vi "niDTS WLAN Tx Test UTIL Parameters to DUT Parameters.vi"(7 "Parameters":T1={"Standard"=enum."802.11 n HT", "DSSS Data Rate (Mbps)"=enum."1", "OFDM Data Rate (Mbps)"=enum."54", "MCS Index"=7, "N spatial streams"=1, "Chains"=[TRUE, FALSE, FALSE, FALSE], "BandWidth (Hz)"=enum."20 MHz", "Channel"=0, "Gard Interval"=enum."SHORT", "FEC Coding"=enum."LDPC", "Dut Tx Power"=1.0, "16 symbols"=TRUE, "payload length bytes"=1500, "idle interval"=0.0001, "External Attenuation"=[0.0, 0.0, 0.0, 0.0], "Acquisition Parameters "={"Acquisition Length Mode"=enum."AUTO", "Acquisition Length (s)"=0.00015, "Auto Level"=FALSE}, "TXP Measurement Parameters"={"TXP Power Enable"=TRUE, "TXP Averages"=3}, "ModAcc Measurement Paramaters"={"ModAcc Enable"=FALSE, "Header Detection"=enum."MANUAL", "Averages"=3, "Amplitude Tracking"=FALSE, "Channel Tracking"=FALSE, "Time Tracking"=TRUE, "Phase Tracking"=enum."NONE", "Clock Offset Est"=FALSE, "Impairments Est"=FALSE, "CFO Estimation"=enum."PAMBLE"}, "ModAcc DSSS Paramaters"={"DC Offset Compensation"=TRUE, "Equalization"=TRUE, "Phase Tracking"=TRUE, "Chip Start Location"=0, "Max Chips Used"=16, "Pulse Shaping FilterType"=enum."GAUSSIAN", "Pulse Shaping Filter Coefficient"=0.35}, "SEM Measurement Parameters"={"SEM Enable"=TRUE, "SEM Averages"=3, "Auto Span Enable"=TRUE, "Frequency Span (Hz)"=66000000.0, "Measurement Type"=enum."Standard", "Mask Frequencies (Hz)"=[], "Mask Power Offsets (dB)"=[]}, "OBW Measurement Parameters"={"OBW Enable"=FALSE, "OBW Averages"=3}, "DSSS Power Ramp"={"Power Ramp Enable"=FALSE, "Averages"=3, "Thresholds"={"Up Low (%)"=10.0, "Down Low (%)"=10.0, "Up High (%)"=90.0, "Down High (%)"=90.0}}, "Enable Traces"=FALSE} {"DSSS Power Ramp"."Thresholds"."Down High (%)" min=0.0 max=100.0 step=1.0; "DSSS Power Ramp"."Thresholds"."Up High (%)" min=0.0 max=100.0 step=1.0; "DSSS Power Ramp"."Thresholds"."Down Low (%)" min=0.0 max=100.0 step=1.0; "DSSS Power Ramp"."Thresholds"."Up Low (%)" min=0.0 max=100.0 step=1.0; "Acquisition Parameters"."Acquisition Length (s)" format="%#_6p"; "SEM Measurement Parameters"."Frequency Span (Hz)" format="%#_6p"; "idle interval" format="%_3p"}) -> (8 "TV Parameters(DataType)":T16={"WLAN Type"=enum."b - 1 Mbps", "Bandwidth (Hz)"=enum."20 MHz", "Channel"=0, "Guard Interval"=enum."LONG", "FEC Coding"=enum."LDPC", "Power (dBm)"=0.0, "Payload Length (bytes)"=1500, "16 Symbols"=TRUE, "Chains"=[TRUE, FALSE, FALSE, FALSE]})   [LabVIEW 2015, in "niDTS WLAN.lvlib"]
uses:
  niDTS WLAN.lvlib
  Includes/niDTS WLAN DUT INC Parameters.ctl
  Includes/niDTS WLAN INC Type.ctl
  Includes/niDTS WLAN INC CH BW.ctl
  Includes/niDTS WLAN INC GI.ctl
  Includes/niDTS WLAN INC FEC Coding.ctl
  Includes/niDTS WLAN Tx Test INC Parameters.ctl
  Includes/niDTS WLAN INC Standard.ctl
  Includes/niDTS WLAN INC DSSS Data Rate.ctl
  Includes/niDTS WLAN INC OFDM Data Rate.ctl
  Includes/niDTS WLAN DUT INC Acquisition Parameters.ctl
  Includes/niDTS WLAN INC TXP Measurement Parameters.ctl
  Includes/niDTS WLAN INC ModAcc Measurement Parameters.ctl
  Includes/niDTS WLAN INC DSSS ModAcc Measurement Parameters.ctl
  Includes/niDTS WLAN INC Pulse Shaping Filter Type.ctl
  Includes/niDTS WLAN INC SEM Measurement Parameters.ctl
  Includes/niDTS WLAN INC OBW Measurement Parameters.ctl
  Includes/niDTS WLAN INC DSSS Power Ramp Parameters.ctl
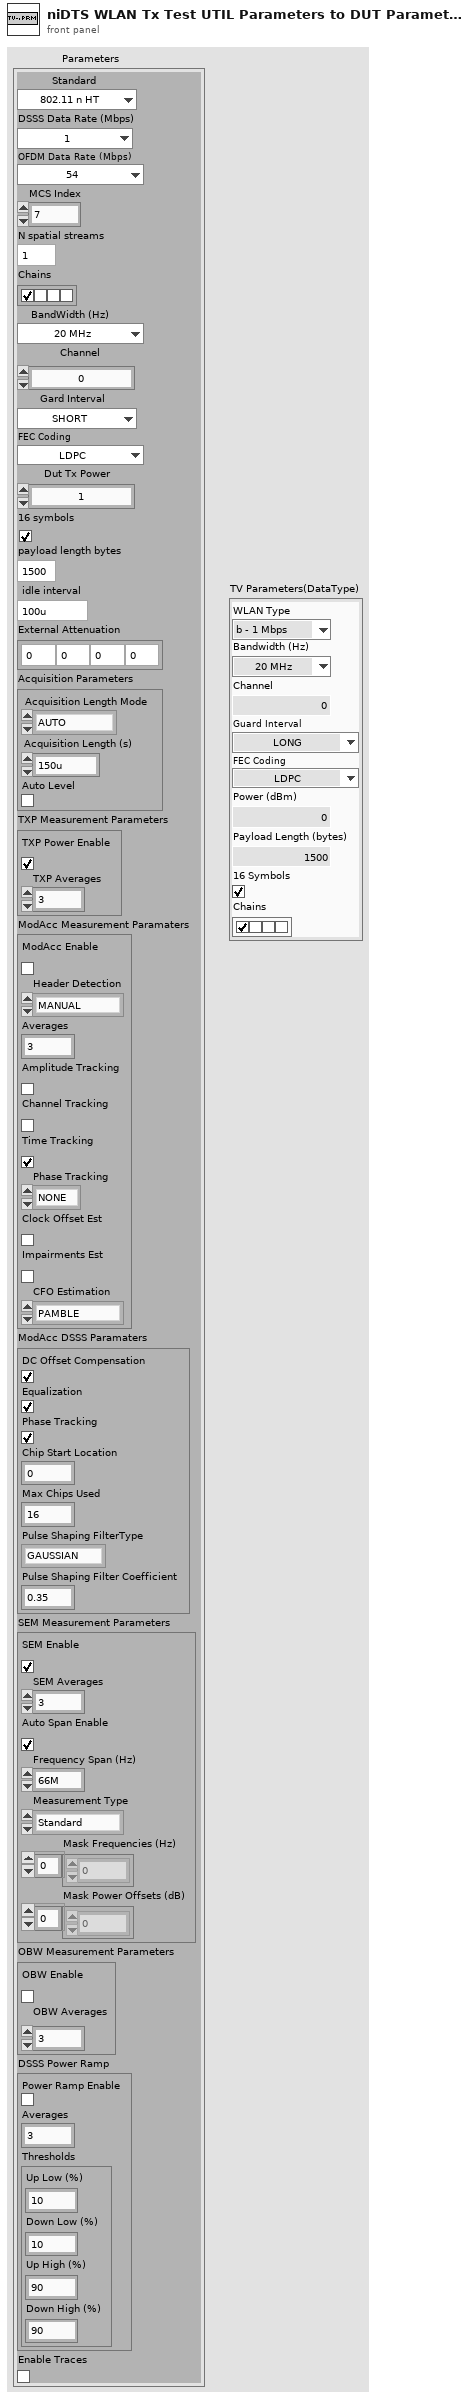
[diagram p1: front panel]
types:
  T1 = typedef "niDTS WLAN.lvlib/niDTS WLAN Tx Test INC Parameters.ctl" = cluster{"Standard":T2, "DSSS Data Rate (Mbps)":T3, "OFDM Data Rate (Mbps)":T4, "MCS Index":i32, "N spatial streams":i32, "Chains":bool[], "BandWidth (Hz)":T5, "Channel":i32, "Gard Interval":T6, "FEC Coding":T7, "Dut Tx Power":dbl, "16 symbols":bool, "payload length bytes":i32, "idle interval":dbl, "External Attenuation":dbl[], "Acquisition Parameters ":T8, "TXP Measurement Parameters":T9, "ModAcc Measurement Paramaters":T10, "ModAcc DSSS Paramaters":T11, "SEM Measurement Parameters":T13, "OBW Measurement Parameters":T14, "DSSS Power Ramp":T15, "Enable Traces":bool}
  T2 = typedef "niDTS WLAN.lvlib/niDTS WLAN INC Standard.ctl" = enum16{"802.11 b DSSS", "802.11 a/g OFDM", "802.11 n HT", "802.11 ac VHT"}
  T3 = typedef "niDTS WLAN.lvlib/niDTS WLAN INC DSSS Data Rate.ctl" = enum16{"1", "2", "5.5", "11"}
  T4 = typedef "niDTS WLAN.lvlib/niDTS WLAN INC OFDM Data Rate.ctl" = enum16{"6", "9", "12", "18", "24", "36", "48", "54"}
  T5 = typedef "niDTS WLAN.lvlib/niDTS WLAN INC CH BW.ctl" = enum16{"20 MHz", "40 MHz", "80 MHz", "160 MHz"}
  T6 = typedef "niDTS WLAN.lvlib/niDTS WLAN INC GI.ctl" = enum16{"LONG", "SHORT"}
  T7 = typedef "niDTS WLAN.lvlib/niDTS WLAN INC FEC Coding.ctl" = enum16{"BCC", "LDPC"}
  T8 = typedef "niDTS WLAN.lvlib/niDTS WLAN DUT INC Acquisition Parameters.ctl" = cluster{"Acquisition Length Mode":enum16{"AUTO", "MANUAL"}, "Acquisition Length (s)":dbl, "Auto Level":bool}
  T9 = typedef "niDTS WLAN.lvlib/niDTS WLAN INC TXP Measurement Parameters.ctl" = cluster{"TXP Power Enable":bool, "TXP Averages":i32}
  T10 = typedef "niDTS WLAN.lvlib/niDTS WLAN INC ModAcc Measurement Parameters.ctl" = cluster{"ModAcc Enable":bool, "Header Detection":enum16{"MANUAL", "FIRST", "ALL"}, "Averages":i32, "Amplitude Tracking":bool, "Channel Tracking":bool, "Time Tracking":bool, "Phase Tracking":enum16{"NONE", "STANDARD", "CSF", "INSTANT"}, "Clock Offset Est":bool, "Impairments Est":bool, "CFO Estimation":enum16{"PAMBLE", "PDATA"}}
  T11 = typedef "niDTS WLAN.lvlib/niDTS WLAN INC DSSS ModAcc Measurement Parameters.ctl" = cluster{"DC Offset Compensation":bool, "Equalization":bool, "Phase Tracking":bool, "Chip Start Location":i16, "Max Chips Used":i16, "Pulse Shaping FilterType":T12, "Pulse Shaping Filter Coefficient":dbl}
  T12 = typedef "niDTS WLAN.lvlib/niDTS WLAN INC Pulse Shaping Filter Type.ctl" = enum16{"NONE", "RCOSINE", "RRCOSINE", "GAUSSIAN"}
  T13 = typedef "niDTS WLAN.lvlib/niDTS WLAN INC SEM Measurement Parameters.ctl" = cluster{"SEM Enable":bool, "SEM Averages":i32, "Auto Span Enable":bool, "Frequency Span (Hz)":dbl, "Measurement Type":enum16{"Standard", "Legacy", "Custom"}, "Mask Frequencies (Hz)":dbl[], "Mask Power Offsets (dB)":dbl[]}
  T14 = typedef "niDTS WLAN.lvlib/niDTS WLAN INC OBW Measurement Parameters.ctl" = cluster{"OBW Enable":bool, "OBW Averages":i32}
  T15 = typedef "niDTS WLAN.lvlib/niDTS WLAN INC DSSS Power Ramp Parameters.ctl" = cluster{"Power Ramp Enable":bool, "Averages":i32, "Thresholds":cluster{"Up Low (%)":dbl, "Down Low (%)":dbl, "Up High (%)":dbl, "Down High (%)":dbl}}
  T16 = typedef "niDTS WLAN.lvlib/niDTS WLAN DUT INC Parameters.ctl" = cluster{"WLAN Type":T17, "Bandwidth (Hz)":T5, "Channel":i32, "Guard Interval":T6, "FEC Coding":T7, "Power (dBm)":dbl, "Payload Length (bytes)":i32, "16 Symbols":bool, "Chains":bool[]}
  T17 = typedef "niDTS WLAN.lvlib/niDTS WLAN INC Type.ctl" = enum16{"b - 1 Mbps", "b - 2 Mbps", "b - 5.5 Mbps", "b - 11 Mbps", "ag - 6 Mbps", "ag - 9 Mbps", "ag - 12 Mbps", "ag - 18 Mbps", "ag - 24 Mbps", "ag - 36 Mbps", "ag - 48 Mbps", "ag - 54 Mbps", "n - MCS0", "n - MCS1", "n - MCS2", "n - MCS3", "n - MCS4", "n - MCS5", "n - MCS6", "n - MCS7", "n - MCS8", "n - MCS9", "n - MCS10", "n - MCS11", "n - MCS12", "n - MCS13", "n - MCS14", "n - MCS15", "n - MCS16", "n - MCS17", "n - MCS18", "n - MCS19", "n - MCS20", "n - MCS21", "n - MCS22", "n - MCS23", "n - MCS24", "n - MCS25", "n - MCS26", "n - MCS27", "n - MCS28", "n - MCS29", "n - MCS30", "n - MCS31", "ac - MCS0 -1", "ac - MCS1 -1", "ac - MCS2 -1", "ac - MCS3 -1", "ac - MCS4 -1", "ac - MCS5 -1", "ac - MCS6 -1", "ac - MCS7 -1", "ac - MCS8 -1", "ac - MCS9 -1", "ac - MCS0 -2", "ac - MCS1 -2", "ac - MCS2 -2", "ac - MCS3 -2", "ac - MCS4 -2", "ac - MCS5 -2", "ac - MCS6 -2", "ac - MCS7 -2", "ac - MCS8 -2", "ac - MCS9 -2", "ac - MCS0 -3", "ac - MCS1 -3", "ac - MCS2 -3", "ac - MCS3 -3", "ac - MCS4 -3", "ac - MCS5 -3", "ac - MCS6 -3", "ac - MCS7 -3", "ac - MCS8 -3", "ac - MCS9 -3", "ac - MCS0 -4", "ac - MCS1 -4", "ac - MCS2 -4", "ac - MCS3 -4", "ac - MCS4 -4", "ac - MCS5 -4", "ac - MCS6 -4", "ac - MCS7 -4", "ac - MCS8 -4", "ac - MCS9 -4"}
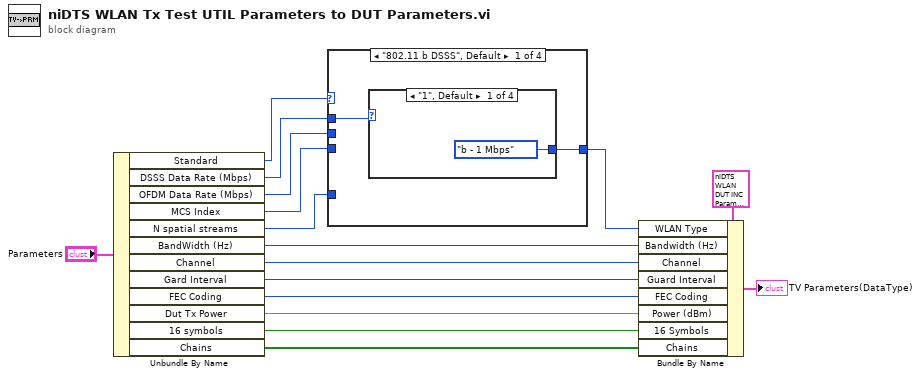
[diagram p0: block diagram]
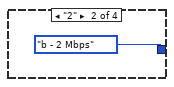
[diagram p2: hidden frame]
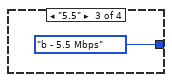
[diagram p3: hidden frame]
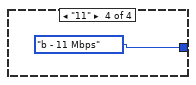
[diagram p4: hidden frame]
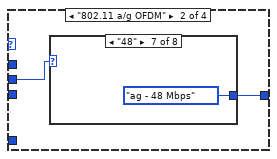
[diagram p5: hidden frame]
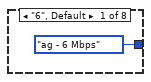
[diagram p6: hidden frame]
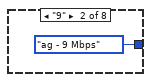
[diagram p7: hidden frame]
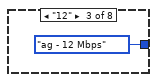
[diagram p8: hidden frame]
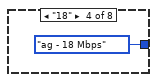
[diagram p9: hidden frame]
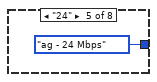
[diagram p10: hidden frame]
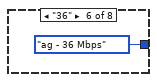
[diagram p11: hidden frame]
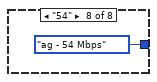
[diagram p12: hidden frame]
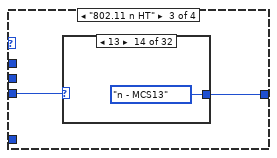
[diagram p13: hidden frame]
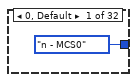
[diagram p14: hidden frame]
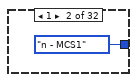
[diagram p15: hidden frame]
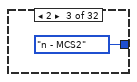
[diagram p16: hidden frame]
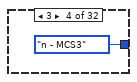
[diagram p17: hidden frame]
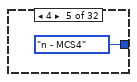
[diagram p18: hidden frame]
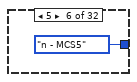
[diagram p19: hidden frame]
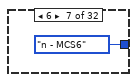
[diagram p20: hidden frame]
diagram:
  n1 = Unbundle By Name("Parameters") -> ("Standard"=w5:T2, "DSSS Data Rate (Mbps)"=w6:T3, "OFDM Data Rate (Mbps)"=w12:T4, "MCS Index"=w11:i32, "N spatial streams"=w7:i32, "BandWidth (Hz)"=w10:T5, "Channel"=w9:i32, "Gard Interval"=w15:T6, "FEC Coding"=w1:T7, "Dut Tx Power"=w8:dbl, "16 symbols"=w4:bool, "Chains"=w3:bool[])
  n2 = case shown="\"802.11 b DSSS\", Default" w5 {
    tunnel: w11 -> [_ _ w34 w73]
    tunnel: w12 -> [_ w24 _ _]
    tunnel: [w18 w23 w33 w69] -> w13
    tunnel: w7 -> [_ _ _ w68]
    tunnel: w6 -> [w17 _ _ _]
    frame "802.11 b DSSS", Default {
      n3 = case shown="\"1\", Default" w17 {
        tunnel: [niDTS_WLAN_INC_Type."b - 1 Mbps" ("WLAN Type 2") niDTS_WLAN_INC_Type."b - 2 Mbps" ("WLAN Type 2") niDTS_WLAN_INC_Type."b - 5.5 Mbps" ("WLAN Type 2") niDTS_WLAN_INC_Type."b - 11 Mbps" ("WLAN Type 2")] -> w18
        frame "1", Default {
        }
        frame "2" {
        }
        frame "5.5" {
        }
        frame "11" {
        }
      }
    }
    frame "802.11 a/g OFDM" {
      n4 = case shown="\"48\"" w24 {
        tunnel: [niDTS_WLAN_INC_Type."ag - 6 Mbps" ("WLAN Type 2") niDTS_WLAN_INC_Type."ag - 9 Mbps" ("WLAN Type 2") niDTS_WLAN_INC_Type."ag - 12 Mbps" ("WLAN Type 2") niDTS_WLAN_INC_Type."ag - 18 Mbps" ("WLAN Type 2") niDTS_WLAN_INC_Type."ag - 24 Mbps" ("WLAN Type 2") niDTS_WLAN_INC_Type."ag - 36 Mbps" ("WLAN Type 2") niDTS_WLAN_INC_Type."ag - 48 Mbps" ("WLAN Type 2") niDTS_WLAN_INC_Type."ag - 54 Mbps" ("WLAN Type 2")] -> w23
        frame "6", Default {
        }
        frame "9" {
        }
        frame "12" {
        }
        frame "18" {
        }
        frame "24" {
        }
        frame "36" {
        }
        frame "48" {
        }
        frame "54" {
        }
      }
    }
    frame "802.11 n HT" {
      n5 = case shown="13" w34 {
        tunnel: [niDTS_WLAN_INC_Type."n - MCS0" ("WLAN Type 2") niDTS_WLAN_INC_Type."n - MCS1" ("WLAN Type 2") niDTS_WLAN_INC_Type."n - MCS2" ("WLAN Type 2") niDTS_WLAN_INC_Type."n - MCS3" ("WLAN Type 2") niDTS_WLAN_INC_Type."n - MCS4" ("WLAN Type 2") niDTS_WLAN_INC_Type."n - MCS5" ("WLAN Type 2") niDTS_WLAN_INC_Type."n - MCS6" ("WLAN Type 2") niDTS_WLAN_INC_Type."n - MCS7" ("WLAN Type 2") niDTS_WLAN_INC_Type."n - MCS8" ("WLAN Type 2") niDTS_WLAN_INC_Type."n - MCS9" ("WLAN Type 2") niDTS_WLAN_INC_Type."n - MCS10" ("WLAN Type 2") niDTS_WLAN_INC_Type."n - MCS11" ("WLAN Type 2") niDTS_WLAN_INC_Type."n - MCS12" ("WLAN Type 2") niDTS_WLAN_INC_Type."n - MCS13" ("WLAN Type 2") niDTS_WLAN_INC_Type."n - MCS14" ("WLAN Type 2") niDTS_WLAN_INC_Type."n - MCS15" ("WLAN Type 2") niDTS_WLAN_INC_Type."n - MCS16" ("WLAN Type 2") niDTS_WLAN_INC_Type."n - MCS17" ("WLAN Type 2") niDTS_WLAN_INC_Type."n - MCS18" ("WLAN Type 2") niDTS_WLAN_INC_Type."n - MCS19" ("WLAN Type 2") niDTS_WLAN_INC_Type."n - MCS20" ("WLAN Type 2") niDTS_WLAN_INC_Type."n - MCS21" ("WLAN Type 2") niDTS_WLAN_INC_Type."n - MCS22" ("WLAN Type 2") niDTS_WLAN_INC_Type."n - MCS23" ("WLAN Type 2") niDTS_WLAN_INC_Type."n - MCS24" ("WLAN Type 2") niDTS_WLAN_INC_Type."n - MCS25" ("WLAN Type 2") niDTS_WLAN_INC_Type."n - MCS26" ("WLAN Type 2") niDTS_WLAN_INC_Type."n - MCS27" ("WLAN Type 2") niDTS_WLAN_INC_Type."n - MCS28" ("WLAN Type 2") niDTS_WLAN_INC_Type."n - MCS29" ("WLAN Type 2") niDTS_WLAN_INC_Type."n - MCS30" ("WLAN Type 2") niDTS_WLAN_INC_Type."n - MCS31" ("WLAN Type 2")] -> w33
        frame 0, Default {
        }
        frame 1 {
        }
        frame 2 {
        }
        frame 3 {
        }
        frame 4 {
        }
        frame 5 {
        }
        frame 6 {
        }
        frame 7 {
        }
        frame 8 {
        }
        frame 9 {
        }
        frame 10 {
        }
        frame 11 {
        }
        frame 12 {
        }
        frame 13 {
        }
        frame 14 {
        }
        frame 15 {
        }
        frame 16 {
        }
        frame 17 {
        }
        frame 18 {
        }
        frame 19 {
        }
        frame 20 {
        }
        frame 21 {
        }
        frame 22 {
        }
        frame 23 {
        }
        frame 24 {
        }
        frame 25 {
        }
        frame 26 {
        }
        frame 27 {
        }
        frame 28 {
        }
        frame 29 {
        }
        frame 30 {
        }
        frame 31 {
        }
      }
    }
    frame "802.11 ac VHT" {
      n6 = case shown="0, Default" w73 {
        tunnel: [niDTS_WLAN_INC_Type."ac - MCS0 -1" ("WLAN Type 2") niDTS_WLAN_INC_Type."ac - MCS1 -1" ("WLAN Type 2") niDTS_WLAN_INC_Type."ac - MCS2 -1" ("WLAN Type 2") niDTS_WLAN_INC_Type."ac - MCS3 -1" ("WLAN Type 2") niDTS_WLAN_INC_Type."ac - MCS4 -1" ("WLAN Type 2") niDTS_WLAN_INC_Type."ac - MCS5 -1" ("WLAN Type 2") niDTS_WLAN_INC_Type."ac - MCS6 -1" ("WLAN Type 2") niDTS_WLAN_INC_Type."ac - MCS7 -1" ("WLAN Type 2") niDTS_WLAN_INC_Type."ac - MCS8 -1" ("WLAN Type 2") niDTS_WLAN_INC_Type."ac - MCS9 -1" ("WLAN Type 2")] -> w72
        frame 0, Default {
        }
        frame 1 {
        }
        frame 2 {
        }
        frame 3 {
        }
        frame 4 {
        }
        frame 5 {
        }
        frame 6 {
        }
        frame 7 {
        }
        frame 8 {
        }
        frame 9 {
        }
      }
      n7 = Decrement(x=w68) -> (x-1=w67:i32)
      n8 = Multiply(x=w67, y=10) -> (x*y=w70:i32)
      n9 = Add(x=w72, y=w70) -> (x+y=w69:i32)
    }
  }
  n10 = Bundle By Name(cluster=T16 {"WLAN Type"=enum."ac - MCS7 -1", "Bandwidth (Hz)"=enum."20 MHz", "Channel"=36, "Guard Interval"=enum."LONG", "FEC Coding"=enum."LDPC", "Power (dBm)"=0.0, "Payload Length (bytes)"=1500, "16 Symbols"=TRUE, "Chains"=[TRUE, FALSE, FALSE, FALSE]} ("output cluster"), "WLAN Type"=w13, "Bandwidth (Hz)"=w10, "Channel"=w9, "Guard Interval"=w15, "FEC Coding"=w1, "Power (dBm)"=w8, "16 Symbols"=w4, "Chains"=w3) -> (→"TV Parameters(DataType)":T16)
